vi "Read from File.vi"(8 "error in (no error)":errorcluster, 10 "INI Ref":T1, 11 "Macro Step in":refnum<class "Macro Step.lvclass">) -> (0 "error out":errorcluster, 2 "INI Ref out":T1, 3 "Macro Step out":refnum<class "Macro Step.lvclass">)   [LabVIEW 2020, in "MacroAssert.lvlib" / "Macro Step.lvclass"]
uses:
  Macro Step.lvclass
  C:/Users/acasalen/Documents/LabVIEW Data/Projects/MacroAssert/source/Classes/Step/Step.lvclass
  Step/Step.lvclass
  <vilib>/Utility/config.llb/NI_LVConfig.lvlib
  <vilib>/Utility/config.llb/Read Key (I32).vi
  MacroAssert.lvlib
  <vilib>/Utility/config.llb/Config Data RefNum.ctl
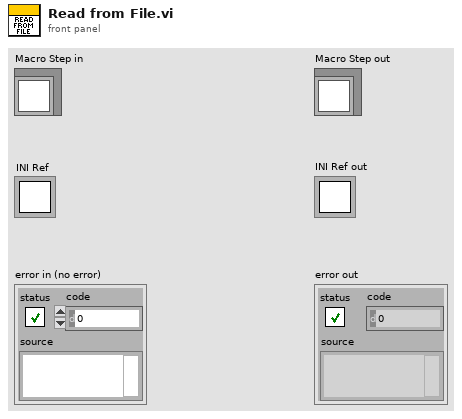
[diagram p1: front panel]
types:
  T1 = typedef "NI_LVConfig.lvlib/Config Data RefNum.ctl" = refnum<k1>
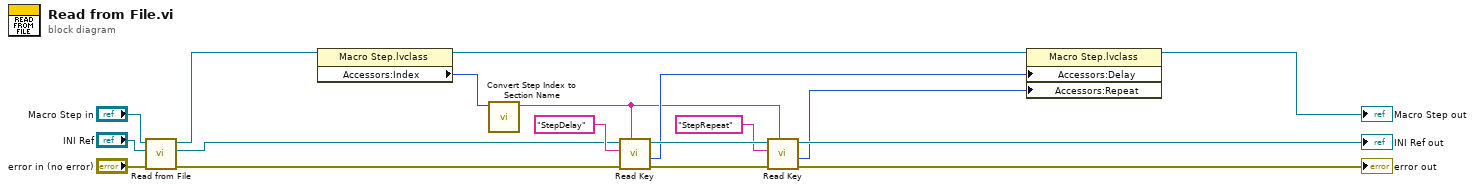
[diagram p0: block diagram]
diagram:
  n1 = call-parent "Read from File.vi"("error in (no error)"="error in (no error)", "INI Ref"="INI Ref", "Step in"="Macro Step in") -> ("error out"=w2:errorcluster, "INI Ref out"=w1:T1, "Step out"=w3:refnum<class "Macro Step.lvclass">)  [unwired: 6 in]
  n2 = property class="Macro Step.lvclass"(reference=w3) -> (reference out=w7:refnum<class "Macro Step.lvclass">, "Accessors:Index"=w6:i32)  [unwired: 1 in, 1 out]
  n3 = call "Convert Step Index to Section Name.vi"("Step Index"=w6) -> ("Section Name"=w5:string)  [unwired: 10 in]
  n4 = call-poly <vilib>:"Read Key.vi"("section"=w5, "error in (no error)"=w2, "key"="StepDelay", "refnum"=w1) -> ("error out"=w14:errorcluster, "value"=w10:i32, "refnum out"=w13:T1)  [unwired: 4 in, 1 out]
  n5 = call-poly <vilib>:"Read Key.vi"("section"=w5, "error in (no error)"=w14, "key"="StepRepeat", "refnum"=w13) -> ("error out"=→"error out":errorcluster, "value"=w8:i32, "refnum out"=→"INI Ref out":T1)  [unwired: 4 in, 1 out]
  n6 = property class="Macro Step.lvclass"(reference=w7, "Accessors:Delay"=w10, "Accessors:Repeat"=w8) -> (reference out=→"Macro Step out":refnum<class "Macro Step.lvclass">)  [unwired: 1 in, 1 out]
